vi "ziExample-NodeDocumentation.vi"() -> ()   [LabVIEW 2009]
doc: "Control a Zurich Instruments device via a LabOne Labview API.\nExample from the Getting Started guide: An array of parameters is element-wise set. The procedure is a useful building block that ensures to always measure with the same settings.\n\n© Zurich Instruments AG, www.zhinst.com"
uses:
  <instrlib>/Zurich Instruments LabOne/Zurich Instruments LabOne.lvlib
panel:
  in  "stop":bool
  in  "Flags (None)":T1
  out "Doc":T2(array[cluster])
  in  "Path":string
  out "Error Out":errorcluster
  in  "Address":string="DEV"
  out "Selected Device":string
  # "ziExample-NodeDocumentation.vi\nRequirements:  UHFLI or MFLI see block diagram for VI description"
  # "Tested Devices:\n- UHFLI\n- MFLI"
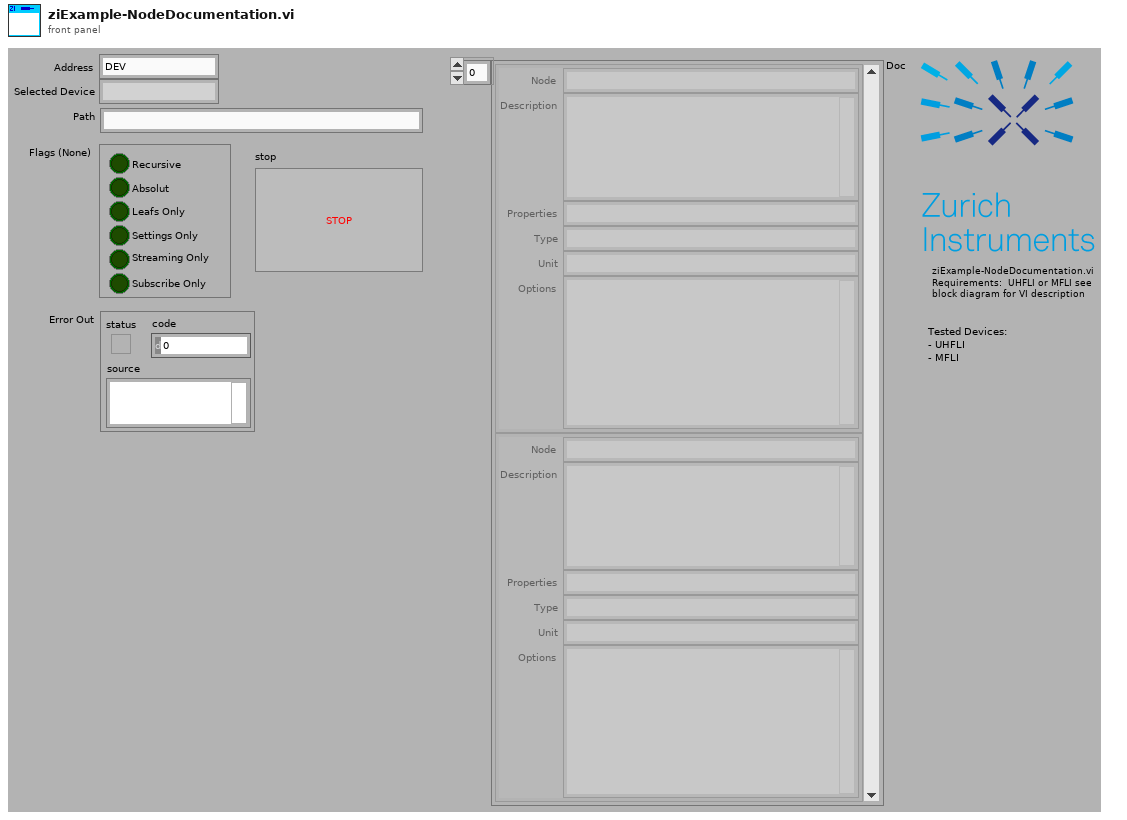
[diagram p1: front panel]
types:
  T1 = cluster{"Recursive":bool, "Absolut":bool, "Leafs Only":bool, "Settings Only":bool, "Streaming Only":bool, "Subscribe Only":bool}
  T2 = cluster{"Node":string, "Description":string, "Properties":string, "Type":string, "Unit":string, "Options":string}[]
  T3 = typedef "Zurich Instruments LabOne.lvlib/ziTypeHandle.ctl" = cluster{"handleValid":bool, "Conn":u64, "Path Prefix":string, "Handle":u64, "Connected":bool, "Clockbase(s)":dbl}
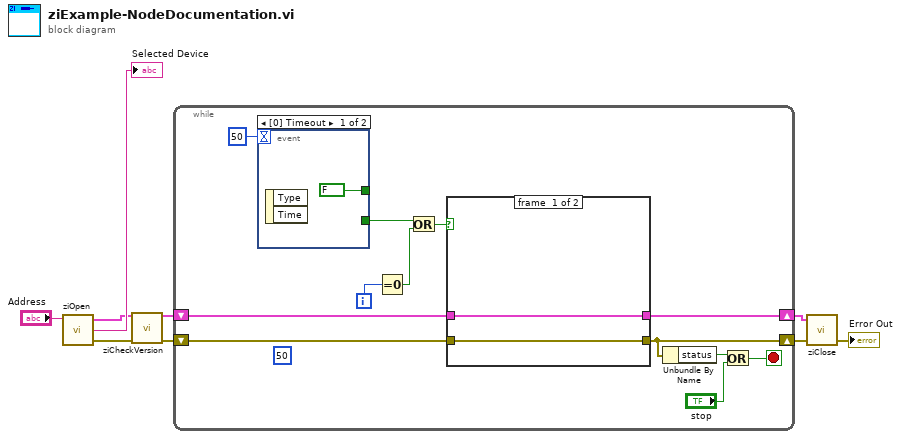
[diagram p0: block diagram]
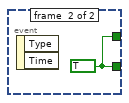
[diagram p2: hidden frame]
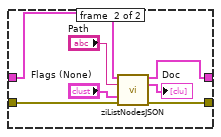
[diagram p3: hidden frame]
diagram:
  n1 = call <instrlib>:"ziOpen.vi"("Address"="Address") -> ("Error Out"=w5:errorcluster, "Selected Device"=→"Selected Device":string, "HandleOut"=w6:T3)  [unwired: 1 in, 2 out]
  n2 = call <instrlib>:"ziCheckVersion.vi"("Handle In"=w6, "Error In"=w5) -> ("Handle Out"=w4:T3, "Error Out"=w3:errorcluster)  [unwired: 11 in, 1 out]
  n3 = while {
    shift-right: [w19] -> w1
    shift-left: w4 -> [w21]
    shift-right: [w18] -> w2
    shift-left: w3 -> [w20]
    i -> [w10]
    stop <- w16 stop-if-true
    (unwired) 50
    n4 = event shown="[0] Timeout" {
      selector: _ -> [_ _]
      dyn-events: _ -> [_ _]
      timeout: 50 -> [_ _]
      tunnel: [FALSE w23] -> _
      tunnel: [_ w23] -> w13
      event #0 {
        n5 = event-data() -> ()  [unwired: 1 in, 2 out]
      }
      event #1 {
        w23 = TRUE
        n6 = event-data() -> ()  [unwired: 1 in, 2 out]
      }
    }
    n7 = Equal To 0?(x=w10) -> (x = 0?=w12:bool)
    n8 = Or(x=w13, y=w12) -> (x .or. y?=w11:bool)
    n9 = case shown="True" w11 {
      tunnel: w21 -> [w25 w32]
      tunnel: w20 -> [w24 w31]
      tunnel: [w25 w30] -> w19
      tunnel: [w24 w29] -> w18
      frame #0 {
      }
      frame #1 {
        n10 = call <instrlib>:"ziListNodesJSON.vi"("Handle In"=w32, "Path (\"\")"="Path", "Flags (None)"="Flags (None)", "Error In"=w31) -> ("Handle Out"=w30:T3, "Doc"=→"Doc":T2, "Error Out"=w29:errorcluster)  [unwired: 9 in]
      }
    }
    n11 = Unbundle By Name(w18) -> ("status"=w17:bool)
    n12 = Or(x=w17, y="stop") -> (x .or. y?=w16:bool)
  }
  n13 = call <instrlib>:"ziClose.vi"("Error In"=w2, "Handle In"=w1) -> ("Error Out"=→"Error Out":errorcluster)  [unwired: 2 in, 1 out]
